vi "GFITS_responseToQ.vi"(8 "error in":errorcluster, 11 "queue name":string) -> (0 "error out":errorcluster)   [LabVIEW 2016]
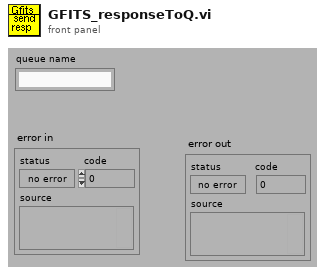
[diagram p1: front panel]
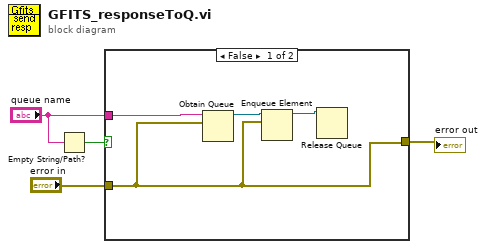
[diagram p0: block diagram]
diagram:
  n1 = Empty String/Path?(string/path="queue name") -> (empty?=w3:bool)
  n2 = case shown="False" w3 {
    tunnel: "queue name" -> [w8 _]
    tunnel: "error in" -> [w6 w9]
    tunnel: [w6 w9] -> w1
    frame False {
      n3 = Obtain Queue(name (unnamed)=w8, element data type=w6) -> (queue out=w7:refnum<queue>)  [unwired: 3 in, 2 out]
      n4 = Enqueue Element(queue=w7, element=w6) -> (queue out=w5:refnum<queue>)  [unwired: 1 in, 3 out]
      n5 = Release Queue(queue=w5) -> ()  [unwired: 1 in, 4 out]
    }
    frame True {
    }
  }
  "error out" <- w1
